vi "PID.vi"(2 "Kd":dbl, 3 "Ki":dbl, 4 "Kp":dbl, 5 "error(t-2)":dbl, 6 "error (t-1)":dbl, 7 "error total(t-1)":dbl) -> (0 "Error Total (t)":dbl, 1 "Sinyal Kontrol":dbl)   [LabVIEW 2016]
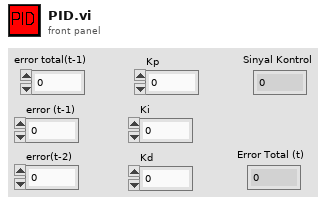
[diagram p1: front panel]
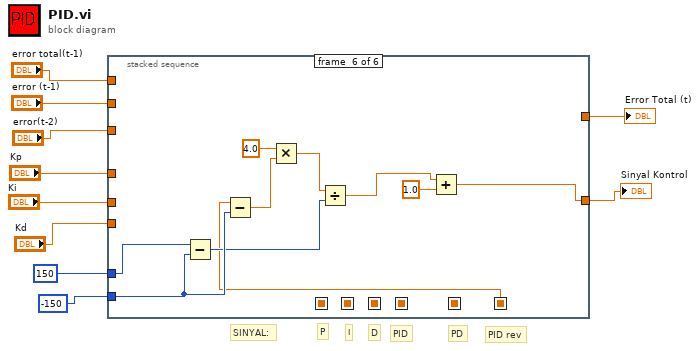
[diagram p0: block diagram]
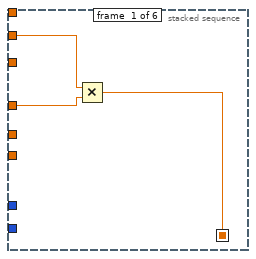
[diagram p2: hidden frame]
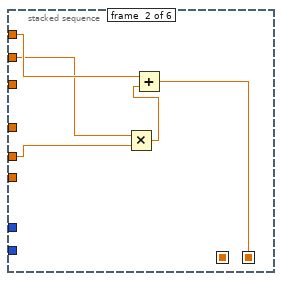
[diagram p3: hidden frame]
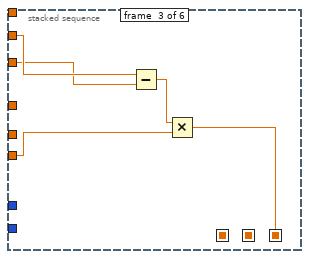
[diagram p4: hidden frame]
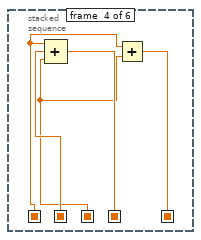
[diagram p5: hidden frame]
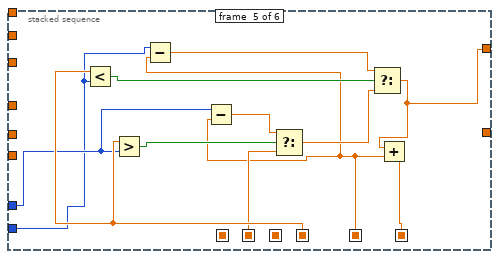
[diagram p6: hidden frame]
diagram:
  # "SINYAL:"
  # "PID rev"
  # "PD"
  # "PID"
  # "D"
  # "I"
  # "P"
  n1 = stacked-sequence {
    seq-local: [w11 _ _ _ _ _] -> [_ _ _ w25 _ _]
    seq-local: [_ w14 _ _ _ _] -> [_ _ _ w26 w36 _]
    seq-local: [_ _ w19 _ _ _] -> [_ _ _ w24 _ _]
    seq-local: [_ _ _ w27 _ _] -> [_ _ _ _ w38 _]
    seq-local: [_ _ _ w28 _ _] -> [_ _ _ _ w31 _]
    seq-local: [_ _ _ _ w40 _] -> [_ _ _ _ _ w41]
    tunnel: "error total(t-1)" -> [_ w18 _ _ _ _]
    tunnel: "error (t-1)" -> [w13 w17 w23 _ _ _]
    tunnel: "error(t-2)" -> [_ _ w22 _ _ _]
    tunnel: "Kp" -> [w12 _ _ _ _ _]
    tunnel: "Ki" -> [_ w16 _ _ _ _]
    tunnel: "Kd" -> [_ _ w21 _ _ _]
    tunnel: [_ _ _ _ w29 _] -> w4
    tunnel: [_ _ _ _ _ w42] -> w3
    tunnel: 150 -> [_ _ _ _ w37 w50]
    tunnel: -150 -> [_ _ _ _ w30 w49]
    frame #0 {
      n2 = Multiply(x=w13, y=w12) -> (x*y=w11:dbl)
    }
    frame #1 {
      n3 = Multiply(x=w17, y=w16) -> (x*y=w15:dbl)
      n4 = Add(x=w18, y=w15) -> (x+y=w14:dbl)
    }
    frame #2 {
      n5 = Subtract(x=w23, y=w22) -> (x-y=w20:dbl)
      n6 = Multiply(x=w20, y=w21) -> (x*y=w19:dbl)
    }
    frame #3 {
      n7 = Compound Arithmetic op=ADD(w25, w26, w24) -> (w27:dbl)
      n8 = Add(x=w25, y=w24) -> (x+y=w28:dbl)
    }
    frame #4 {
      n9 = Less?(x=w38, y=w30) -> (x < y?=w39:bool)
      n10 = Greater?(x=w38, y=w37) -> (0:w35:bool)
      n11 = Subtract(x=w30, y=w31) -> (x-y=w32:dbl)
      n12 = Subtract(x=w37, y=w31) -> (x-y=w34:dbl)
      n13 = Select(t=w34, s=w35, f=w36) -> (s? t:f=w33:dbl)
      n14 = Select(t=w32, s=w39, f=w33) -> (s? t:f=w29:dbl)
      n15 = Add(x=w29, y=w31) -> (x+y=w40:dbl)
    }
    frame #5 {
      n16 = Subtract(x=w50, y=w49) -> (x-y=w48:i32)
      n17 = Subtract(x=w41, y=w49) -> (x-y=w45:dbl)
      n18 = Multiply(x=4.0, y=w45) -> (x*y=w47:dbl)
      n19 = Divide(x=w47, y=w48) -> (x/y=w44:dbl)
      n20 = Add(x=w44, y=1.0) -> (x+y=w42:dbl)
    }
  }
  "Sinyal Kontrol" <- w3
  "Error Total (t)" <- w4
